vi "Get Response Coefficients.vi"(8 "error in (no error)":errorcluster, 11 "Sinusoidal Fit in":refnum<class "Sinusoidal Fit.lvclass">) -> (0 "error out":errorcluster, 2 "Coefficients":T1 {"Freq" format="%#.2f"; "Offset" format="%.3f"; "Gain" format="%.2f"; "Phase" format="%.1f"}, 3 "Sinusoidal Fit out":refnum<class "Sinusoidal Fit.lvclass">)   [LabVIEW 2016, in "Sinusoidal Fit.lvclass"]
uses:
  Sinusoidal Fit.lvclass
  gain and phase/Typedef - Sinusoidal Fit Coefficients.ctl
  Sinusoidal Fit.lvclass/Sinusoidal Fit.ctl
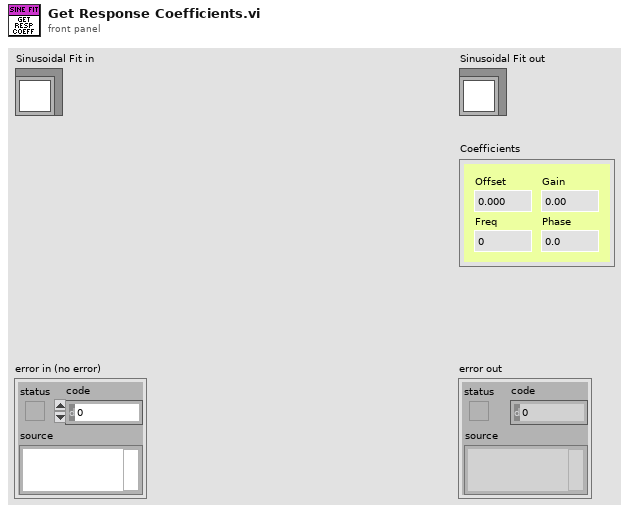
[diagram p1: front panel]
types:
  T1 = typedef "Typedef - Sinusoidal Fit Coefficients.ctl" = cluster{"Offset":dbl, "Gain":dbl, "Phase":dbl, "Freq":dbl}
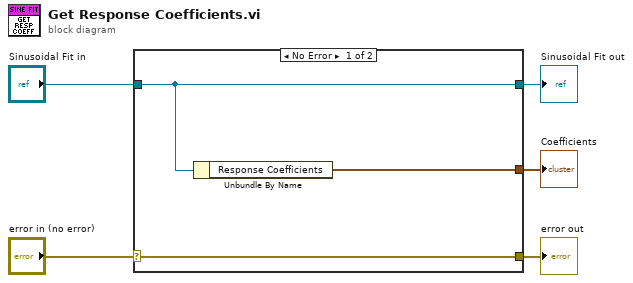
[diagram p0: block diagram]
diagram:
  n1 = case shown="No Error" "error in (no error)" {
    selector: "error in (no error)" -> [w8 w9]
    tunnel: [w8 w9] -> w4
    tunnel: [w7 w10] -> w2
    tunnel: "Sinusoidal Fit in" -> [w7 w10]
    tunnel: [w6 _] -> w1
    frame No Error {
      n2 = Unbundle By Name(w7) -> ("Response Coefficients"=w6:T1)
    }
    frame Error {
    }
  }
  "error out" <- w4
  "Sinusoidal Fit out" <- w2
  "Coefficients" <- w1
